vi "Get Service Descriptor.vi"(8 "error in":errorcluster, 11 "measurement plugin in":refnum<class "Automotive Ethernet Bus Monitor.lvclass">) -> (0 "error out":errorcluster, 2 "service descriptor":T1, 3 "measurement plugin out":refnum<class "Automotive Ethernet Bus Monitor.lvclass">)   [LabVIEW 2025, in "Automotive Ethernet Bus Monitor.lvclass"]
uses:
  Automotive Ethernet Bus Monitor.lvclass
  <vilib>/Plug-In SDKs/Measurements/Helpers/TypeDefs/Service Descriptor.ctl
  <vilib>/Plug-In SDKs/Measurements/Helpers/TypeDefs/Measurement Details.ctl
  <vilib>/Plug-In SDKs/Measurements/Helpers/TypeDefs/Measurement Annotation.ctl
  Automotive Ethernet Bus Monitor.lvclass/Automotive Ethernet Bus Monitor.ctl
  <vilib>/Plug-In SDKs/Measurements/NI Measurement Plug-In SDK.lvlib
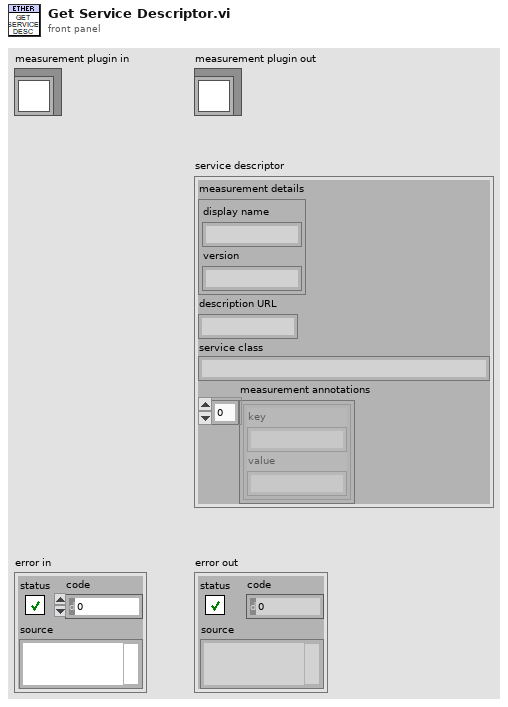
[diagram p1: front panel]
types:
  T1 = typedef "NI Measurement Plug-In SDK.lvlib/Service Descriptor.ctl" = cluster{"measurement details":T2, "description URL":string, "service class":string, "measurement annotations":T3[]}
  T2 = typedef "NI Measurement Plug-In SDK.lvlib/Measurement Details.ctl" = cluster{"display name":string, "version":string}
  T3 = typedef "NI Measurement Plug-In SDK.lvlib/Measurement Annotation.ctl" = cluster{"key":string, "value":string}
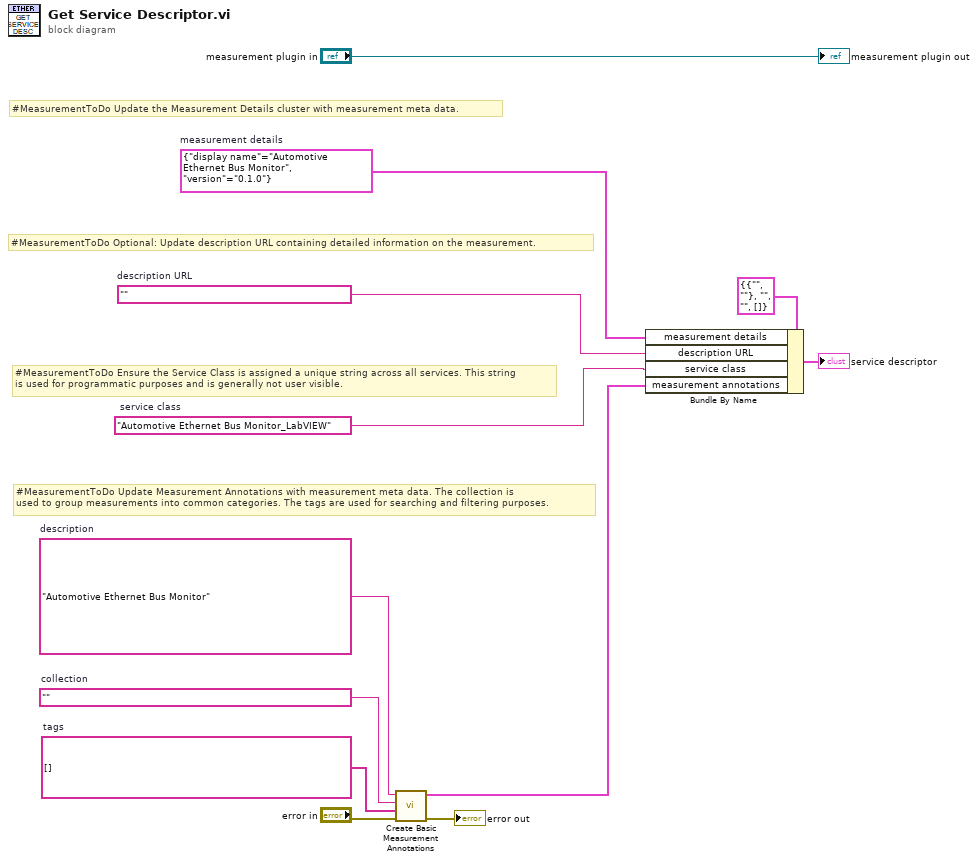
[diagram p0: block diagram]
diagram:
  w8 = ""  # description URL
  w10 = string[] []  # tags
  w11 = ""  # collection
  w12 = "Automotive Ethernet Bus Monitor"  # description
  w9 = T2 {"display name"="Automotive Ethernet Bus Monitor", "version"="0.1.0"}  # measurement details
  w7 = "Automotive Ethernet Bus Monitor_LabVIEW"  # service class
  # "#MeasurementToDo Optional: Update description URL containing detailed information on the measurement."
  # "#MeasurementToDo Update Measurement Annotations with measurement meta data. The collection is\nused to group measurements into common categories. The tags are used for searching and filtering purposes."
  # "#MeasurementToDo Ensure the Service Class is assigned a unique string across all services. This string\nis used for programmatic purposes and is generally not user visible."
  # "#MeasurementToDo Update the Measurement Details cluster with measurement meta data."
  n1 = call <vilib>:"Create Basic Measurement Annotations.vi"("error in"="error in", "tags"=w10, "collection"=w11, "description"=w12) -> ("error out"=→"error out":errorcluster, "measurement annotations"=w6:T3[])  [unwired: 6 in]
  n2 = Bundle By Name(cluster=T1 {"measurement details"={"display name"="", "version"=""}, "description URL"="", "service class"="", "measurement annotations"=[]} ("service descriptor"), "measurement details"=w9, "description URL"=w8, "service class"=w7, "measurement annotations"=w6) -> (→"service descriptor":T1)
  "measurement plugin out" <- "measurement plugin in"
